vi "HeaderAction.vi"(0 "InstrClass":refnum<class "BNC845.lvclass"> caption="DNL_LabVIEW Object in", 11 "error in (no error)":errorcluster caption="entrée d'erreur (pas d'erreur)") -> (4 "InstrClassOut":refnum<class "BNC845.lvclass"> caption="DNL_LabVIEW Object out", 6 "DataNames":string[](array[string]), 8 "Instr Name":string, 10 "HeaderString":string, 13 "ArrDisplayNames":string[](array[string]), 14 "DisplayNames":string[](array[string]), 15 "error out":errorcluster caption="sortie d'erreur")   [LabVIEW 2019, in "BNC845.lvclass"]
uses:
  BNC845.lvclass
  C:/Programmes Labview/LabScanV1A/DevicesClass/BaseDevice/BaseDevice.lvclass
  BNC845.lvclass/BNC845.ctl
  BaseDevice/BaseDevice.lvclass
  <instrlib>/Berkeley Nucleonics 845/Berkeley Nucleonics 845.lvlib
panel:
  in  "FUnits":u16(ring) caption="Units" items=["Hz", "MHz", "GHz"]
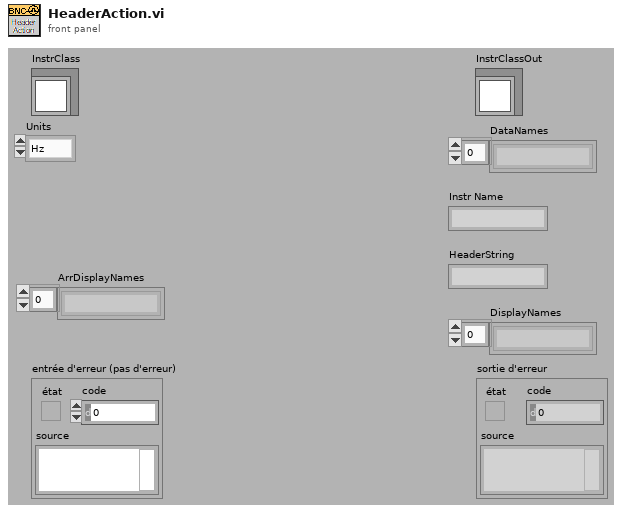
[diagram p1: front panel]
types:
  T1 = typedef "BNC845.lvclass/BNC845_Func.ctl" = enum16{"SetPower (dBm)", "SetFrequency (Hz)"}
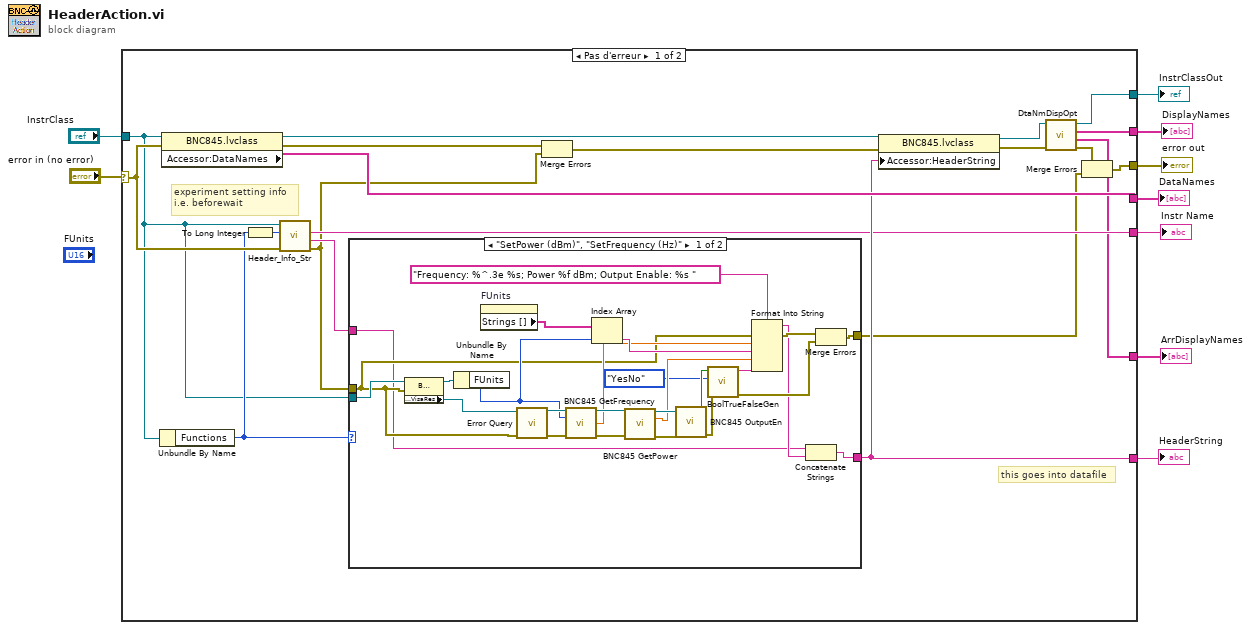
[diagram p0: block diagram]
diagram:
  n1 = case shown="Pas d'erreur" "error in (no error)" {
    selector: "error in (no error)" -> [w18 w58]
    tunnel: [w26 _] -> w8
    tunnel: [w29 _] -> w7
    tunnel: "InstrClass" -> [w13 w59]
    tunnel: [w11 w58] -> w5
    tunnel: [w23 w59] -> w3
    tunnel: [w20 _] -> w4
    tunnel: [w21 _] -> w2
    tunnel: [w14 _] -> w1
    frame No Error {
      # "this goes into datafile"
      # "experiment setting info\ni.e. beforewait"
      n2 = Unbundle By Name(w13) -> ("Functions"=w16:T1)
      n3 = property class="BNC845.lvclass"(reference=w13, error in=w18) -> (reference out=w28:refnum<class "BNC845.lvclass">, error out=w27:errorcluster, "Accessor:DataNames"=w29:string[])
      n4 = To Long Integer(number=w16) -> (32bit integer=w15:i32)
      n5 = call-dynamic "Header_Info_Str.vi"("error in (no error)"=w18, "Functions"=w15, "DefaultDev in"=w13) -> ("error out"=w12:errorcluster, "HdrInfoStr"=w19:string, "InstrumentName"=w20:string)  [unwired: 5 in, 1 out]
      n6 = case shown="\"SetPower (dBm)\", \"SetFrequency (Hz)\"" w16 {
        tunnel: [w31 w57] -> w26
        tunnel: w19 -> [w30 w57]
        tunnel: w13 -> [w47 _]
        tunnel: w12 -> [w41 w56]
        tunnel: [w34 w56] -> w10
        frame "SetPower (dBm)", "SetFrequency (Hz)" {
          n7 = property class="BNC845.lvclass"(reference=w47, error in=w41) -> (reference out=w48:refnum<class "BNC845.lvclass">, "Accessor:VisaRes"=w49:refnum<visa-resource-name>)  [unwired: 1 out]
          n8 = Unbundle By Name(w48) -> ("FUnits"=w45:u16)
          n9 = property on="FUnits" class="MDér (strict)"() -> ("Strings []"=w46:string[])  [unwired: 2 in, 2 out]
          n10 = call <instrlib>:"Error Query.vi"("VISA resource name"=w49, "error in (no error)"=w41) -> ("VISA resource name out"=w54:refnum<visa-resource-name>, "error out"=w55:errorcluster)  [unwired: 10 in, 2 out]
          n11 = call <instrlib>:"BNC845 GetFrequency.vi"("VISA Rsrc"=w54, "FUnits"=w45, "error in (no error)"=w55) -> ("VISA Rsrc Out"=w52:refnum<visa-resource-name>, "Frequency (Units)"=w42:dbl, "error out"=w53:errorcluster)  [unwired: 9 in, 1 out]
          n12 = Index Array(array=w46, index=w45) -> (element=w43:string)
          n13 = call <instrlib>:"BNC845 GetPower.vi"("VISA Rsrc"=w52, "error in (no error)"=w53) -> ("VISA Rsrc Out"=w50:refnum<visa-resource-name>, "Power (dBm)"=w40:dbl, "error out"=w51:errorcluster)  [unwired: 11 in]
          n14 = call <instrlib>:"BNC845 OutputEn.vi"("VISA Rsrc"=w50, "error in (no error)"=w51) -> ("Enabled"=w39:bool, "error out"=w38:errorcluster)  [unwired: 11 in, 1 out]
          n15 = call <userlib>:"BoolTrueFalseGen.vi"("Error in"=w38, "Énum"=enum16{"TrueFalse", "YesNo", "OnOff"}."YesNo", "Bool"=w39) -> ("Error out"=w33:errorcluster, "TrueFalse"=w37:string)  [unwired: 6 in]
          n16 = Format Into String(format string="Frequency: %^.3e %s; Power %f dBm; Output Enable: %s " ("chaîne de format"), error in=w41, w42, w43, w40, w37) -> (resulting string=w32:string, error out=w35:errorcluster)  [unwired: 1 in]
          n17 = Concatenate Strings(w30, w32) -> (w31:string)
          n18 = Merge Errors(w35, w33) -> (w34:errorcluster)
        }
        frame Default {
        }
      }
      n19 = Merge Errors(w27, w12) -> (w17:errorcluster)
      n20 = property class="BNC845.lvclass"(reference=w28, error in=w17, "Accessor:HeaderString"=w26) -> (reference out=w22:refnum<class "BNC845.lvclass">, error out=w25:errorcluster)
      n21 = call "DtaNmDispOpt.vi"("error in (no error)"=w25, "BaseDevice en entrée"=w22) -> ("error out"=w24:errorcluster, "ArrDisplayNames"=w14:string[], "DisplayNames"=w21:string[], "BaseDevice en sortie"=w23:refnum<class "BNC845.lvclass">)  [unwired: 6 in]
      n22 = Merge Errors(w24, w10) -> (w11:errorcluster)
    }
    frame Error {
    }
  }
  "error out" <- w5
  "InstrClassOut" <- w3
  "DataNames" <- w7
  "HeaderString" <- w8
  "Instr Name" <- w4
  "DisplayNames" <- w2
  "ArrDisplayNames" <- w1
